vi "Calc_Line.vi"(9 "end":cluster{"x":dbl, "y":dbl}, 10 "start":cluster{"x":dbl, "y":dbl}) -> (2 "line":cluster{"slope":dbl, "b":dbl, "theta":dbl})   [LabVIEW 2022 SP3]
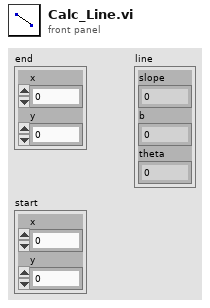
[diagram p1: front panel]
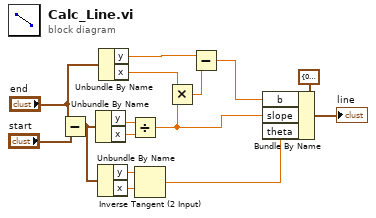
[diagram p0: block diagram]
diagram:
  n1 = Subtract(x="end", y="start") -> (x-y=w2:cluster{"x":dbl, "y":dbl})
  n2 = Unbundle By Name(w2) -> ("y"=w6:dbl, "x"=w5:dbl)
  n3 = Unbundle By Name(w2) -> ("y"=w4:dbl, "x"=w3:dbl)
  n4 = Unbundle By Name("end") -> ("y"=w10:dbl, "x"=w9:dbl)
  n5 = Divide(x=w6, y=w5) -> (x/y=w14:dbl)
  n6 = Inverse Tangent (2 Input)(1:w3, 2:w4) -> (0:w1:dbl)
  n7 = Multiply(x=w9, y=w14) -> (x*y=w11:dbl)
  n8 = Subtract(x=w10, y=w11) -> (x-y=w13:dbl)
  n9 = Bundle By Name(cluster=cluster{"slope":dbl, "b":dbl, "theta":dbl} {"slope"=0.0, "b"=0.0, "theta"=0.0} ("line"), "b"=w13, "slope"=w14, "theta"=w1) -> (→"line":cluster{"slope":dbl, "b":dbl, "theta":dbl})
